vi "dr_dtheta.vi"(1 "Wind Vector":cluster{"Wind R":dbl, "Wind Theta":dbl}, 2 "Goal Angle":dbl, 3 "Boat Angle":dbl) -> (0 "dr/dtheta":dbl)   [LabVIEW 2011]
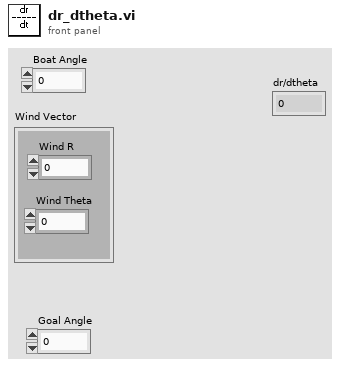
[diagram p1: front panel]
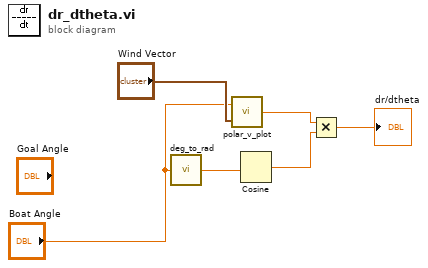
[diagram p0: block diagram]
diagram:
  n1 = call "deg_to_rad.vi"("Degrees"="Boat Angle") -> ("Radians"=w6:dbl)
  n2 = call "polar_v_plot.vi"("Wind Vector"="Wind Vector", "Boat Angle"="Boat Angle") -> ("Velocity"=w4:dbl)
  n3 = Cosine(x=w6) -> (cos(x)=w2:dbl)
  n4 = Multiply(x=w4, y=w2) -> (x*y=→"dr/dtheta":dbl)
